vi "GET_Show.vi"(8 "error in":errorcluster {"code" min=0 max=0}, 11 "Settings.lvclass in":refnum<class "Settings.lvclass">) -> (0 "error out":errorcluster {"code" min=0 max=0}, 1 "Show Terminals?":bool, 3 "Settings.lvclass out":refnum<class "Settings.lvclass">)   [LabVIEW 2020, in "Settings.lvclass"]
uses:
  Settings.lvclass
  Settings.lvclass/Settings.ctl
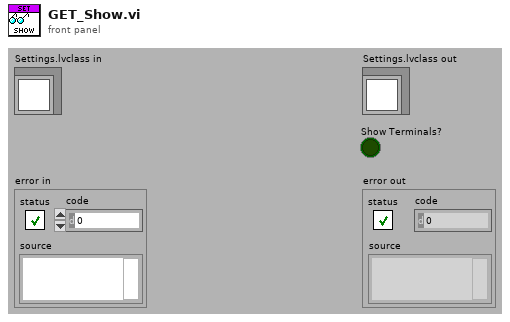
[diagram p1: front panel]
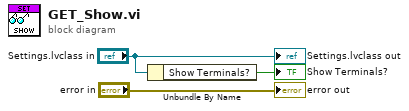
[diagram p0: block diagram]
diagram:
  n1 = Unbundle By Name("Settings.lvclass in") -> ("Show Terminals?"=→"Show Terminals?":bool)
  "error out" <- "error in"
  "Settings.lvclass out" <- "Settings.lvclass in"
